vi "System.Processes.vi"(8 "error in":errorcluster, 10 "Kill":bool, 11 "Process Name":string) -> (0 "error out":errorcluster, 2 "Is Running":bool, 3 "Processes":string[](array[string]))   [LabVIEW 2018]
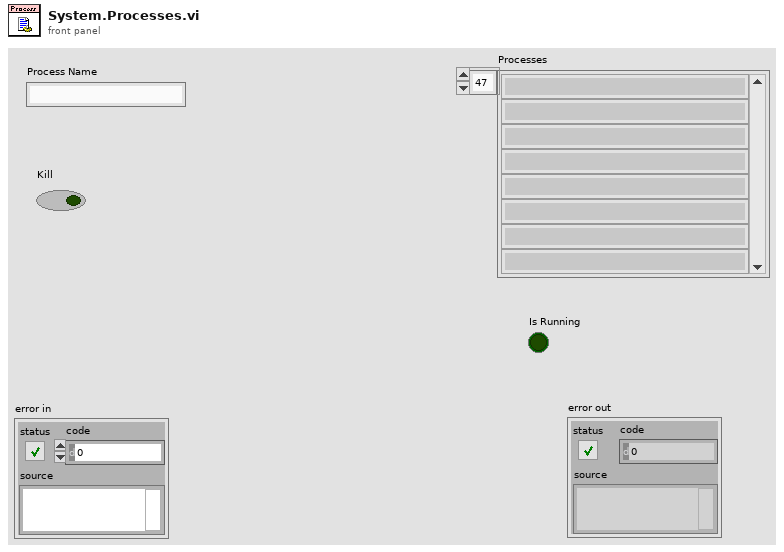
[diagram p1: front panel]
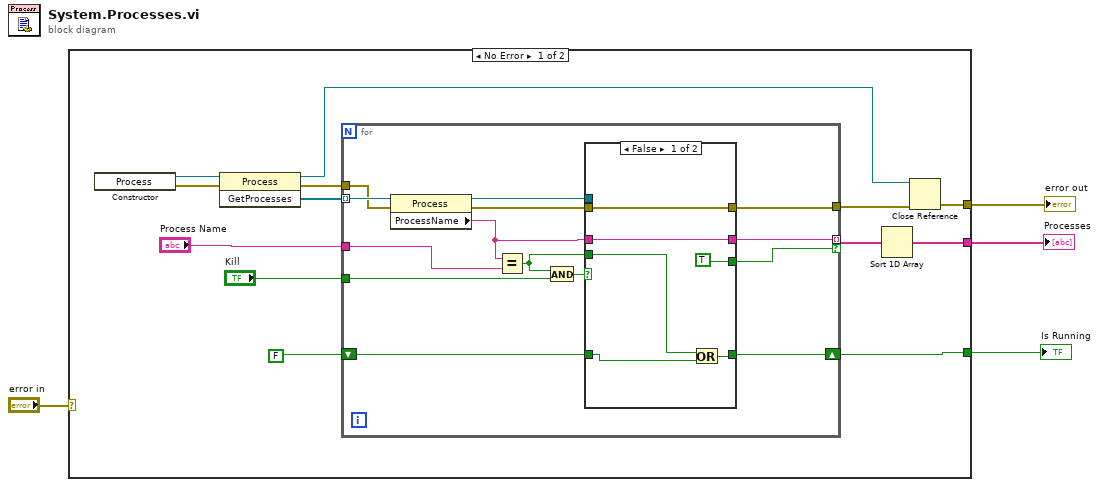
[diagram p0: block diagram]
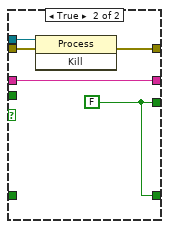
[diagram p2: hidden frame]
diagram:
  n1 = case shown="No Error" "error in" {
    selector: "error in" -> [_ w43]
    tunnel: [w9 w43] -> w4
    tunnel: [w5 _] -> w3
    tunnel: [w7 _] -> w2
    frame No Error {
      n2 = constructor class="Process"() -> (reference out=w17:refnum<k24>, error out=w16:errorcluster)  [unwired: 3 in, 1 out]
      n3 = invoke class="Process" method="GetProcesses"(reference=w17, error in=w16) -> (reference out=w10:refnum<k24>, error out=w13:errorcluster, "GetProcesses"=w14:refnum<k24>[])  [unwired: 1 in]
      n4 = for {
        tunnel: "Process Name" -> [w31]
        tunnel: w14 -> [w30] mode=indexing
        tunnel: w13 -> [w27]
        tunnel: "Kill" -> [w26]
        tunnel: [w23] -> w6 mode=indexing if=w21
        tunnel: [w22] -> w11
        shift-right: [w20] -> w7
        shift-left: FALSE -> [w18]
        n5 = property class="Process"(reference=w30, error in=w27) -> (reference out=w29:refnum<k24>, error out=w28:errorcluster, "ProcessName"=w24:string)
        n6 = Equal?(x=w24, y=w31) -> (x = y?=w19:bool)
        n7 = And(x=w19, y=w26) -> (x .and. y?=w25:bool)
        n8 = case shown="False" w25 {
          tunnel: w29 -> [_ w42]
          tunnel: w28 -> [w35 w41]
          tunnel: w24 -> [w36 w40]
          tunnel: [w36 w40] -> w23
          tunnel: [w35 w39] -> w22
          tunnel: [TRUE w38] -> w21
          tunnel: [w34 w38] -> w20
          tunnel: w19 -> [w33 _]
          tunnel: w18 -> [w32 _]
          frame False {
            n9 = Or(x=w33, y=w32) -> (x .or. y?=w34:bool)
          }
          frame True {
            w38 = FALSE
            n10 = invoke class="Process" method="Kill"(reference=w42, error in=w41) -> (error out=w39:errorcluster)  [unwired: 1 in, 2 out]
          }
        }
      }
      n11 = Sort 1D Array(array=w6) -> (sorted array=w5:string[])
      n12 = Close Reference(reference=w10, error in (no error)=w11) -> (error out=w9:errorcluster)
    }
    frame Error {
    }
  }
  "Is Running" <- w2
  "error out" <- w4
  "Processes" <- w3
